vi "Slave - Data Integrity - Organized.vi"() -> ()   [LabVIEW 2016]
uses:
  <vilib>/Utility/error.llb/DialogType.ctl
  <vilib>/pximc/Initialize Writer Session (DBL).vi
  <vilib>/pximc/Initialize Reader Session (DBL).vi
  <vilib>/pximc/Connect (DBL).vi
  <vilib>/pximc/Acquire Write Region (DBL).vi
  <vilib>/pximc/Acquire Read Region (DBL).vi
  <vilib>/pximc/nipximc.lvlib
  <resource>/objmgr/pximc.rc
panel:
  out "Writer Node 2":T1(graph)
  out "Writer Node 1":T1(graph)
  out "Stopped?":bool=TRUE
  in  "Stop Button":bool
  in  "#Writing Channels Slave 2":i32=2
  in  "#Reading Channels Slave 2":i32=4
  out "Reader Node 1":T1(graph)
  in  "#Reading Channels Slave 1":i32=4
  in  "#Writing Channels Slave 1":i32=2
  out "Reader Node 2":T1(graph)
  in  "Node 1 Reader Connection ID":u16=4
  in  "Reader Interface Node 2":tag="PXIMC2" caption="interface"
  in  "Node 2 Writer Connection ID":u16=3
  in  "Writer Interface Node 2":tag="PXIMC2" caption="interface"
  in  "Node 1 Writer Connection ID":u16=1
  in  "Node 1 Writer Interface":tag="PXIMC2" caption="interface"
  in  "Node 1 Reader Interface":tag="PXIMC2" caption="interface"
  in  "Buffer Size":u64=250000 caption="buffer size"
  in  "Connection Timeout (s)":dbl=60.0 caption="timeout in seconds (-1)"
  in  "Node 1 Reader Connection ID":u16=2
  # "Node 1"
  # "Node 2"
  # "Node 2 => Node 1"
  # "Node 1 => Node 2"
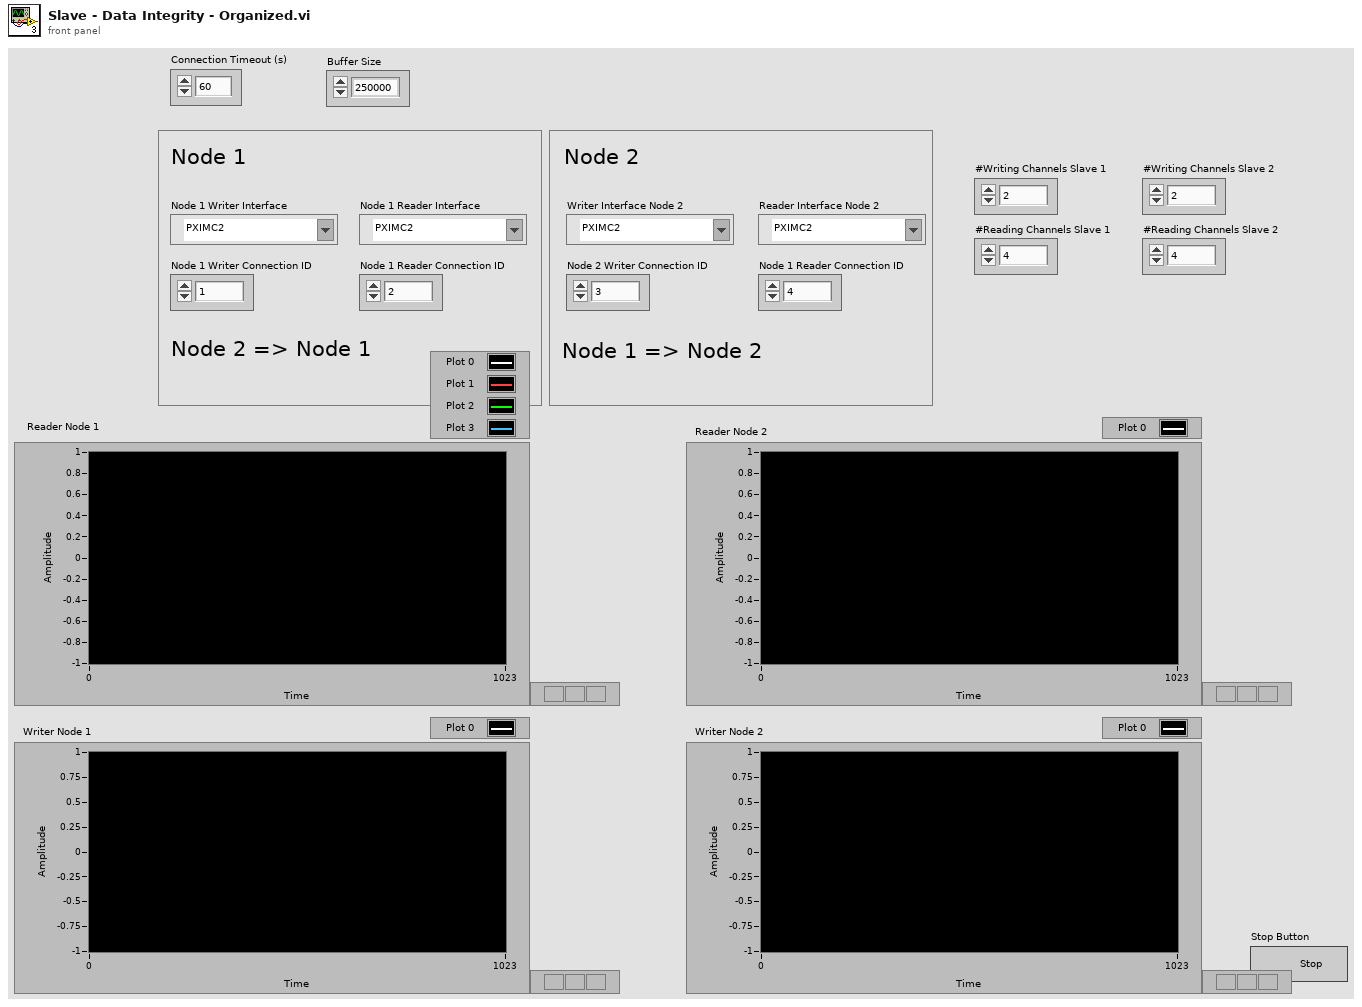
[diagram p1: front panel]
types:
  T1 = cluster{"[0]":dbl, "[1]":dbl, "[2]":dbl, "[3]":dbl, "[4]":dbl, "[5]":dbl, "[6]":dbl, "[7]":dbl, "[8]":dbl}
  T2 = typedef "DialogType.ctl" = u16
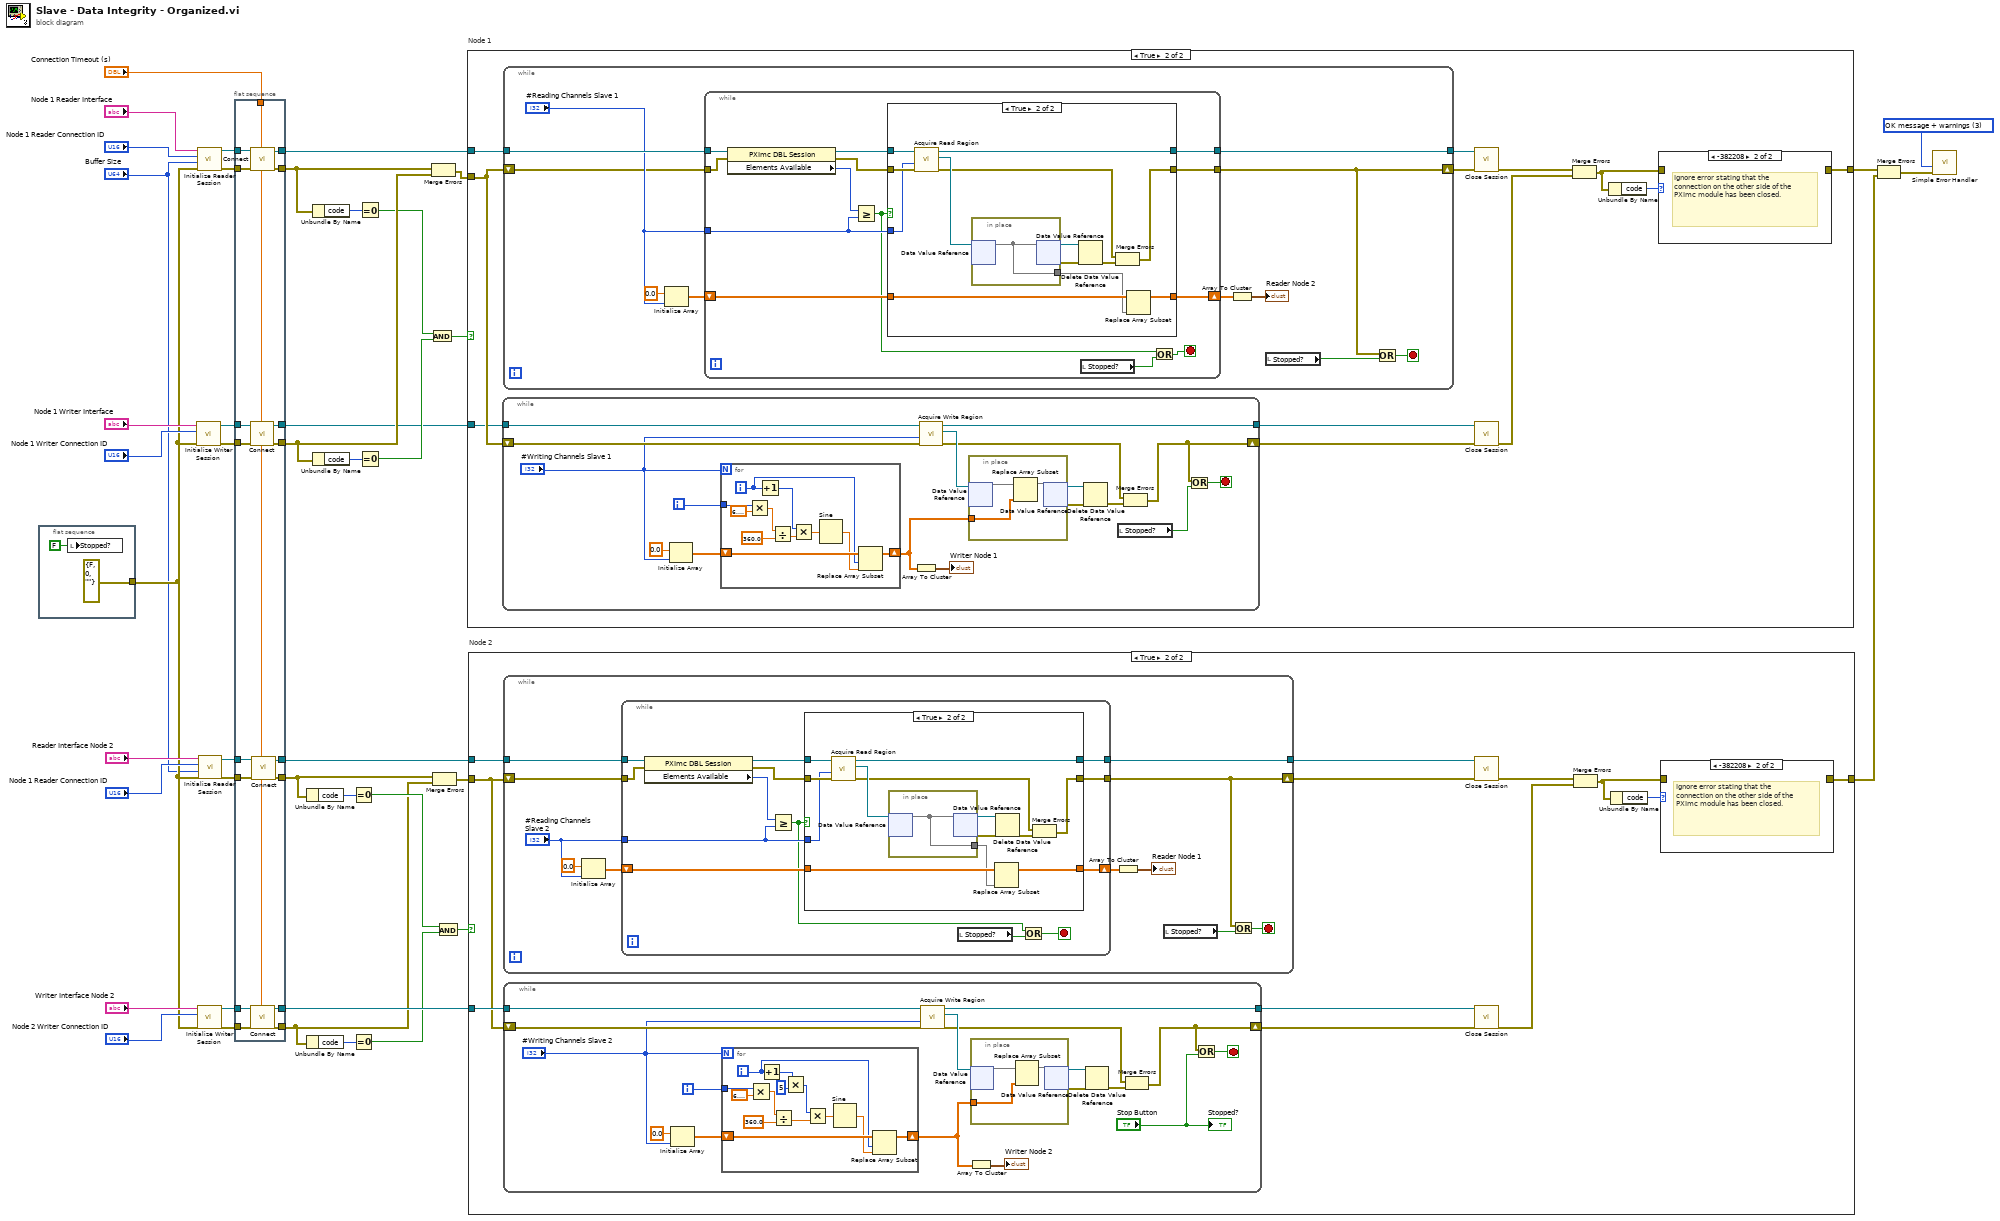
[diagram p0: block diagram]
diagram:
  w37 = T2 3 items=["no dialog", "OK message", "continue or stop message", "OK message + warnings", "continue/stop + warnings"] ("type of dialog (OK msg:1)")
  n1 = flat-sequence {
    tunnel: [errorcluster {"status"=FALSE, "code"=0, "source"=""} ("error constant")] -> w15
    frame #0 {
      n2 = local write "Stopped?"(FALSE ("Stopped?")) -> ()
    }
  }
  n3 = call-poly <vilib>:"Initialize Writer Session.vi"("error in (no error)"=w15, "connection id (1)"="Node 1 Writer Connection ID", "interface"="Node 1 Writer Interface") -> ("error out"=w35:errorcluster, "session out"=w34:refnum<k21>)  [unwired: 7 in]
  n4 = call-poly <vilib>:"Initialize Reader Session.vi"("error in (no error)"=w15, "buffer size"="Buffer Size", "writer's connection id (1)"="Node 1 Reader Connection ID", "interface"="Node 1 Reader Interface") -> ("error out"=w41:errorcluster, "session out"=w42:refnum<k21>)  [unwired: 6 in]
  n5 = call-poly <vilib>:"Initialize Writer Session.vi"("error in (no error)"=w15, "connection id (1)"="Node 2 Writer Connection ID", "interface"="Writer Interface Node 2") -> ("error out"=w22:errorcluster, "session out"=w23:refnum<k21>)  [unwired: 7 in]
  n6 = call-poly <vilib>:"Initialize Reader Session.vi"("error in (no error)"=w15, "buffer size"="Buffer Size", "writer's connection id (1)"="Node 1 Reader Connection ID", "interface"="Reader Interface Node 2") -> ("error out"=w18:errorcluster, "session out"=w17:refnum<k21>)  [unwired: 6 in]
  n7 = flat-sequence {
    tunnel: w42 -> [w62]
    tunnel: w41 -> [w61]
    tunnel: [w60] -> w40
    tunnel: w35 -> [w59]
    tunnel: w34 -> [w58]
    tunnel: [w57] -> w29
    tunnel: [w56] -> w28
    tunnel: "Connection Timeout (s)" -> [w46]
    tunnel: [w55] -> w26
    tunnel: [w54] -> w11
    tunnel: [w53] -> w3
    tunnel: [w52] -> w4
    tunnel: w23 -> [w51]
    tunnel: w22 -> [w50]
    tunnel: [w49] -> w12
    tunnel: w18 -> [w48]
    tunnel: w17 -> [w47]
    frame #0 {
      n8 = call-poly <vilib>:"Connect.vi"("timeout in seconds (-1)"=w46, "error in (no error)"=w59, "session in"=w58) -> ("error out"=w56:errorcluster, "session out"=w55:refnum<k21>)  [unwired: 7 in]
      n9 = call-poly <vilib>:"Connect.vi"("timeout in seconds (-1)"=w46, "error in (no error)"=w61, "session in"=w62) -> ("error out"=w57:errorcluster, "session out"=w60:refnum<k21>)  [unwired: 7 in]
      n10 = call-poly <vilib>:"Connect.vi"("timeout in seconds (-1)"=w46, "error in (no error)"=w50, "session in"=w51) -> ("error out"=w53:errorcluster, "session out"=w54:refnum<k21>)  [unwired: 7 in]
      n11 = call-poly <vilib>:"Connect.vi"("timeout in seconds (-1)"=w46, "error in (no error)"=w48, "session in"=w47) -> ("error out"=w52:errorcluster, "session out"=w49:refnum<k21>)  [unwired: 7 in]
    }
  }
  n12 = Unbundle By Name(w4) -> ("code"=w20:i32)
  n13 = Unbundle By Name(w3) -> ("code"=w25:i32)
  n14 = Unbundle By Name(w29) -> ("code"=w38:i32)
  n15 = Unbundle By Name(w28) -> ("code"=w32:i32)
  n16 = Equal To 0?(x=w20) -> (x = 0?=w6:bool)
  n17 = Equal To 0?(x=w25) -> (x = 0?=w5:bool)
  n18 = Equal To 0?(x=w38) -> (x = 0?=w13:bool)
  n19 = Equal To 0?(x=w32) -> (x = 0?=w31:bool)
  n20 = And(x=w13, y=w31) -> (x .and. y?=w8:bool)
  n21 = Merge Errors(w29, w28) -> (w30:errorcluster)
  n22 = Merge Errors(w4, w3) -> (w2:errorcluster)
  n23 = And(x=w6, y=w5) -> (x .and. y?=w7:bool)
  n24 = case "Node 1" shown="True" w8 {
    tunnel: w40 -> [_ w75]
    tunnel: w30 -> [w63 w74]
    tunnel: w26 -> [_ w73]
    tunnel: [w63 w72] -> w10
    frame False {
    }
    frame True {
      n25 = while {
        tunnel: w73 -> [w85]
        tunnel: [w84] -> w69
        shift-right: [w81] -> w67
        shift-left: w74 -> [w83]
        i -> [w76]
        stop <- w80 stop-if-true
        n26 = Initialize Array(0.0 ("element"), "#Writing Channels Slave 1") -> (w92:dbl[])
        n27 = for {
          N: "#Writing Channels Slave 1" -> [_]
          tunnel: w76 -> [w100]
          shift-right: [w98] -> w77
          shift-left: w92 -> [w99]
          i -> [w96]
          n28 = Multiply(x=w100, y=6.283185307179586) -> (x*y=w103:dbl)
          n29 = Increment(x=w96) -> (x+1=w101:i32)
          n30 = Divide(x=w103, y=360.0) -> (x/y=w105:dbl)
          n31 = Multiply(x=w101, y=w105) -> (x*y=w106:dbl)
          n32 = Sine(x=w106) -> (sin(x)=w97:dbl)
          n33 = Replace Array Subset(array=w99, new element=w97, index=w96) -> (w98:dbl[])
        }
        n34 = Array To Cluster(array=w77) -> (cluster=→"Writer Node 1":T1)
        n35 = call-poly <vilib>:"Acquire Write Region.vi"("error in (no error)"=w83, "number of elements"="#Writing Channels Slave 1", "session in"=w85) -> ("error out"=w86:errorcluster, "write region reference"=w87:refnum<data-value>, "session out"=w84:refnum<k21>)  [unwired: 5 in, 1 out]
        n36 = in-place {
          in-place-border: w77 -> [w93]
          n37 = in-place-dvr #1(w87) -> (w95:dbl[])  [unwired: 1 out]
          n38 = Replace Array Subset(array=w95, new element=w93) -> (w94:dbl[])  [unwired: 1 in]
          n39 = in-place-dvr #1(w94) -> (w88:refnum<data-value>, w90:errorcluster)
        }
        n40 = Delete Data Value Reference(data value reference=w88, error in=w90) -> (error out=w89:errorcluster)  [unwired: 1 out]
        n41 = local read "Stopped?"() -> (w79:bool)
        n42 = Merge Errors(w86, w89) -> (w81:errorcluster)
        n43 = Or(x=w81, y=w79) -> (x .or. y?=w80:bool)
      }
      n44 = while {
        tunnel: [w111] -> w70
        shift-right: [w110] -> w68
        shift-left: w74 -> [w108]
        tunnel: w75 -> [w115]
        stop <- w117 stop-if-true
        n45 = Initialize Array(0.0 ("element"), "#Reading Channels Slave 1") -> (w114:dbl[])
        n46 = while {
          tunnel: w115 -> [w129]
          tunnel: w108 -> [w126]
          tunnel: [w130] -> w110
          tunnel: "#Reading Channels Slave 1" -> [w122]
          shift-right: [w123] -> w109
          shift-left: w114 -> [w124]
          tunnel: [w121] -> w111
          stop <- w118 stop-if-true
          n47 = property class="PXImc DBL Session"(reference=w129, error in=w126) -> (reference out=w127:refnum<k21>, error out=w125:errorcluster, "Elements Available"=w128:u64)
          n48 = Greater Or Equal?(x=w128, y=w122) -> (x >= y?=w120:bool)
          n49 = case shown="True" w120 {
            tunnel: w125 -> [w133 w145]
            tunnel: [w133 w139] -> w130
            tunnel: w127 -> [w131 w144]
            tunnel: w124 -> [w132 w138]
            tunnel: [w132 w136] -> w123
            tunnel: w122 -> [_ w135]
            tunnel: [w131 w134] -> w121
            frame False {
            }
            frame True {
              n50 = call-poly <vilib>:"Acquire Read Region.vi"("error in (no error)"=w145, "number of elements"=w135, "session in"=w144) -> ("error out"=w140:errorcluster, "read region reference"=w146:refnum<data-value>, "session out"=w134:refnum<k21>)  [unwired: 5 in, 1 out]
              n51 = in-place {
                in-place-border: [w147] -> w137
                n52 = in-place-dvr #2(w146) -> (w147:dbl[])  [unwired: 1 out]
                n53 = in-place-dvr #2(w147) -> (w143:refnum<data-value>, w142:errorcluster)
              }
              n54 = Delete Data Value Reference(data value reference=w143, error in=w142) -> (error out=w141:errorcluster)  [unwired: 1 out]
              n55 = Merge Errors(w140, w141) -> (w139:errorcluster)
              n56 = Replace Array Subset(array=w138, new element=w137) -> (w136:dbl[])  [unwired: 1 in]
            }
          }
          n57 = local read "Stopped?"() -> (w119:bool)
          n58 = Or(x=w120, y=w119) -> (x .or. y?=w118:bool)
        }
        n59 = Array To Cluster(array=w109) -> (cluster=→"Reader Node 2":T1)
        n60 = local read "Stopped?"() -> (w107:bool)
        n61 = Or(x=w110, y=w107) -> (x .or. y?=w117:bool)
      }
      n62 = call <vilib>:"Close Session.vi"("error in (no error)"=w68, "session in"=w70) -> ("error out"=w66:errorcluster)  [unwired: 9 in]
      n63 = call <vilib>:"Close Session.vi"("error in (no error)"=w67, "session in"=w69) -> ("error out"=w65:errorcluster)  [unwired: 9 in]
      n64 = Merge Errors(w66, w65) -> (w64:errorcluster)
      n65 = Unbundle By Name(w64) -> ("code"=w71:i32)
      n66 = case shown="-382208" w71 {
        tunnel: w64 -> [w148 _]
        tunnel: [w148 _] -> w72
        frame 0, Default {
        }
        frame -382208 {
          # "Ignore error stating that the connection on the other side of the PXImc module has been closed."
        }
      }
    }
  }
  n67 = case "Node 2" shown="True" w7 {
    tunnel: w12 -> [_ w161]
    tunnel: w11 -> [_ w160]
    tunnel: w2 -> [w149 w151]
    tunnel: [w149 w150] -> w1
    frame False {
    }
    frame True {
      n68 = while {
        tunnel: [w200] -> w158
        shift-right: [w197] -> w157
        shift-left: w151 -> [w198]
        tunnel: w161 -> [w204]
        stop <- w206 stop-if-true
        n69 = Initialize Array(0.0 ("element"), "#Reading Channels Slave 2") -> (w203:dbl[])
        n70 = while {
          tunnel: w204 -> [w218]
          tunnel: w198 -> [w215]
          tunnel: [w219] -> w197
          tunnel: "#Reading Channels Slave 2" -> [w211]
          shift-right: [w212] -> w199
          shift-left: w203 -> [w213]
          tunnel: [w210] -> w200
          stop <- w207 stop-if-true
          n71 = property class="PXImc DBL Session"(reference=w218, error in=w215) -> (reference out=w216:refnum<k21>, error out=w214:errorcluster, "Elements Available"=w217:u64)
          n72 = Greater Or Equal?(x=w217, y=w211) -> (x >= y?=w208:bool)
          n73 = case shown="True" w208 {
            tunnel: w214 -> [w222 w234]
            tunnel: [w222 w228] -> w219
            tunnel: w216 -> [w220 w233]
            tunnel: w213 -> [w221 w227]
            tunnel: [w221 w225] -> w212
            tunnel: w211 -> [_ w224]
            tunnel: [w220 w223] -> w210
            frame False {
            }
            frame True {
              n74 = call-poly <vilib>:"Acquire Read Region.vi"("error in (no error)"=w234, "number of elements"=w224, "session in"=w233) -> ("error out"=w229:errorcluster, "read region reference"=w235:refnum<data-value>, "session out"=w223:refnum<k21>)  [unwired: 5 in, 1 out]
              n75 = in-place {
                in-place-border: [w236] -> w226
                n76 = in-place-dvr #3(w235) -> (w236:dbl[])  [unwired: 1 out]
                n77 = in-place-dvr #3(w236) -> (w232:refnum<data-value>, w231:errorcluster)
              }
              n78 = Replace Array Subset(array=w227, new element=w226) -> (w225:dbl[])  [unwired: 1 in]
              n79 = Delete Data Value Reference(data value reference=w232, error in=w231) -> (error out=w230:errorcluster)  [unwired: 1 out]
              n80 = Merge Errors(w229, w230) -> (w228:errorcluster)
            }
          }
          n81 = local read "Stopped?"() -> (w209:bool)
          n82 = Or(x=w208, y=w209) -> (x .or. y?=w207:bool)
        }
        n83 = Array To Cluster(array=w199) -> (cluster=→"Reader Node 1":T1)
        n84 = local read "Stopped?"() -> (w196:bool)
        n85 = Or(x=w197, y=w196) -> (x .or. y?=w206:bool)
      }
      n86 = while {
        tunnel: w160 -> [w172]
        tunnel: [w171] -> w159
        shift-right: [w168] -> w156
        shift-left: w151 -> [w170]
        i -> [w165]
        stop <- w167 stop-if-true
        n87 = Initialize Array(0.0 ("element"), "#Writing Channels Slave 2") -> (w179:dbl[])
        n88 = for {
          N: "#Writing Channels Slave 2" -> [_]
          tunnel: w165 -> [w190]
          shift-right: [w188] -> w163
          shift-left: w179 -> [w189]
          i -> [w186]
          n89 = Multiply(x=w190, y=6.283185307179586) -> (x*y=w192:dbl)
          n90 = Increment(x=w186) -> (x+1=w185:i32)
          n91 = Divide(x=w192, y=360.0) -> (x/y=w194:dbl)
          n92 = Multiply(x=w185, y=5) -> (x*y=w183:i32)
          n93 = Multiply(x=w183, y=w194) -> (x*y=w195:dbl)
          n94 = Sine(x=w195) -> (sin(x)=w187:dbl)
          n95 = Replace Array Subset(array=w189, new element=w187, index=w186) -> (w188:dbl[])
        }
        n96 = call-poly <vilib>:"Acquire Write Region.vi"("error in (no error)"=w170, "number of elements"="#Writing Channels Slave 2", "session in"=w172) -> ("error out"=w173:errorcluster, "write region reference"=w174:refnum<data-value>, "session out"=w171:refnum<k21>)  [unwired: 5 in, 1 out]
        n97 = Array To Cluster(array=w163) -> (cluster=→"Writer Node 2":T1)
        n98 = in-place {
          in-place-border: w163 -> [w180]
          n99 = in-place-dvr #4(w174) -> (w182:dbl[])  [unwired: 1 out]
          n100 = Replace Array Subset(array=w182, new element=w180) -> (w181:dbl[])  [unwired: 1 in]
          n101 = in-place-dvr #4(w181) -> (w175:refnum<data-value>, w177:errorcluster)
        }
        n102 = Delete Data Value Reference(data value reference=w175, error in=w177) -> (error out=w176:errorcluster)  [unwired: 1 out]
        n103 = Merge Errors(w173, w176) -> (w168:errorcluster)
        n104 = Or(x=w168, y="Stop Button") -> (x .or. y?=w167:bool)
        "Stopped?" <- "Stop Button"
      }
      n105 = call <vilib>:"Close Session.vi"("error in (no error)"=w157, "session in"=w158) -> ("error out"=w153:errorcluster)  [unwired: 9 in]
      n106 = call <vilib>:"Close Session.vi"("error in (no error)"=w156, "session in"=w159) -> ("error out"=w152:errorcluster)  [unwired: 9 in]
      n107 = Merge Errors(w153, w152) -> (w154:errorcluster)
      n108 = Unbundle By Name(w154) -> ("code"=w155:i32)
      n109 = case shown="-382208" w155 {
        tunnel: w154 -> [w162 _]
        tunnel: [w162 _] -> w150
        frame 0, Default {
        }
        frame -382208 {
          # "Ignore error stating that the connection on the other side of the PXImc module has been closed."
        }
      }
    }
  }
  n110 = Merge Errors(w10, w1) -> (w9:errorcluster)
  n111 = call <vilib>:"Simple Error Handler.vi"("type of dialog (OK msg:1)"=w37, "error in (no error)"=w9) -> ()  [unwired: 3 in, 5 out]
